vi "I2C_Read.vi"(8 "error in (no error)":errorcluster, 9 "Read Size":u8=1, 10 "Device Register":T3 items=["WHOAMI"=0, "HW_REV"=1, "FW_VER_MAJOR"=2, "FW_VER_MINOR"=3, "UPDATE_RATE_HZ"=4, "ACCEL_FSR_G"=5, "GYRO_FSR_DPS"=6, "OP_STATUS"=8, "CAL_STATUS"=9, "SELFTEST_STATUS"=10, "SENSOR_STATUS"=16, "TIMESTAMP"=18, "YAW"=22, "PITCH"=24, "ROLL"=26, "HEADING"=28, "FUSED_HEADING"=30, "ALTITUDE_I"=32, "ALTITUDE_D"=34, "LINERA_ACC_X"=36, "LINERA_ACC_Y"=38, "LINERA_ACC_Z"=40, "QUAT_W"=42, "QUAT_X"=44, "QUAT_Y"=46, "QUAT_Z"=48, "MPU_TEMP_C"=50, "GYRO_X"=52, "GYRO_Y"=54, "GYRO_Z"=56, "ACC_X"=58, "ACC_Y"=60, "ACC_Z"=62, "MAG_X"=64, "MAG_Y"=66, "MAG_Z"=68, "PRESSURE_I"=70, "PRESSURE_D"=72, "PRESSURE_TEMP"=74, "YAW_OFFSET"=76, "QUAT_OFFSET_W"=78, "QUAT_OFFSET_X"=80, "QUAT_OFFSET_Y"=82, "QUAT_OFFSET_Z"=84], 11 "I2CDevRef":T1={"DevStatus"={"status"=FALSE, "code"=0, "source"=""}, "Device Address"=0, "Handle"=0, "I2C Bus"=enum."Invalid"} {"Device Address" format="%.0x"}) -> (0 "error out":errorcluster, 2 "navX Data":u8[](array[numeric]), 3 "I2CDevRef":T1={"DevStatus"={"status"=FALSE, "code"=0, "source"=""}, "Device Address"=0, "Handle"=0, "I2C Bus"=enum."Invalid"} {"Device Address" format="%.0x"})   [LabVIEW 2015, in "navX-MXP IMU.lvlib"]
uses:
  navX-MXP IMU.lvlib
  COMMON/TypeDefs/Value TypeDefs/navX Device Registers.ctl
  <vilib>/Rock Robotics/WPI/I2C/WPI_I2CDevRef.ctl
  <vilib>/Rock Robotics/SystemInterfaces/i2clib/i2c_bus.ctl
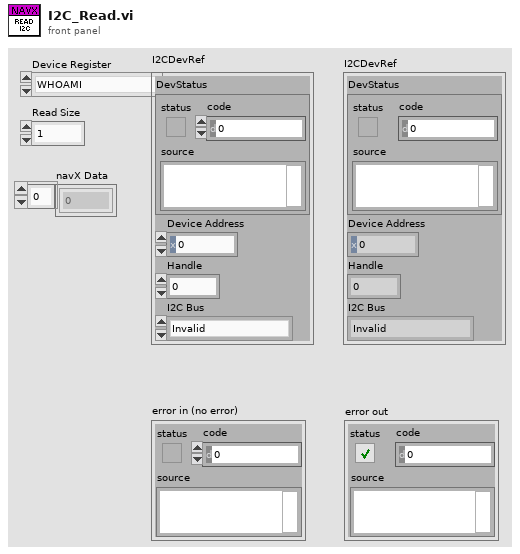
[diagram p1: front panel]
types:
  T1 = typedef "WPI_I2CDevRef.ctl" = cluster{"DevStatus":errorcluster, "Device Address":u8, "Handle":i32, "I2C Bus":T2}
  T2 = typedef "i2c_bus.ctl" = enum16{"I2C On-Board", "I2C MXP", "Invalid"}
  T3 = typedef "navX-MXP IMU.lvlib/navX Device Registers.ctl" = u8
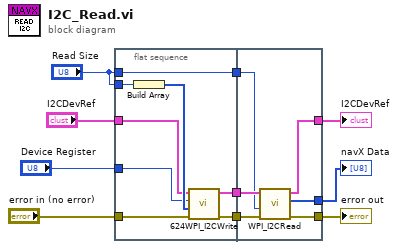
[diagram p0: block diagram]
diagram:
  n1 = flat-sequence {
    tunnel: "Read Size" -> [w15]
    tunnel: "Device Register" -> [w14]
    tunnel: [w17] -> w10
    tunnel: [w16] -> w9
    tunnel: "Read Size" -> [w13]
    tunnel: [w13] -> w5
    tunnel: "I2CDevRef" -> [w12]
    tunnel: "error in (no error)" -> [w11]
    tunnel: [w22] -> w7
    tunnel: [w21] -> w2
    tunnel: [w20] -> w1
    tunnel: w5 -> [w19]
    tunnel: w9 -> [w23]
    tunnel: w10 -> [w24]
    frame #0 {
      n2 = Build Array(w15) -> (w18:u8[])
      n3 = call "624WPI_I2CWrite.vi"("error in (no error)"=w11, "I2CDataToSend"=w18, "I2CRegister"=w14, "I2CDevRef"=w12) -> ("error out"=w16:errorcluster, "I2CDevRef"=w17:T1)  [unwired: 6 in]
    }
    frame #1 {
      n4 = call <vilib>:"WPI_I2CRead.vi"("error in (no error)"=w23, "I2CBytesToRead"=w19, "I2CDevRef"=w24) -> ("error out"=w20:errorcluster, "Data Out"=w22:u8[], "I2CDevRef"=w21:T1)  [unwired: 6 in]
    }
  }
  "navX Data" <- w7
  "I2CDevRef" <- w2
  "error out" <- w1
